vi "Write message.vi"(6 "timeout ms (25000)":i32=25000, 8 "error in":errorcluster, 9 "Value":string, 10 "Message Name":string, 11 "Connection Info":T1) -> (0 "error out":errorcluster, 3 "Connection Info out":T1)   [LabVIEW 2021]
uses:
  Connection Info.ctl
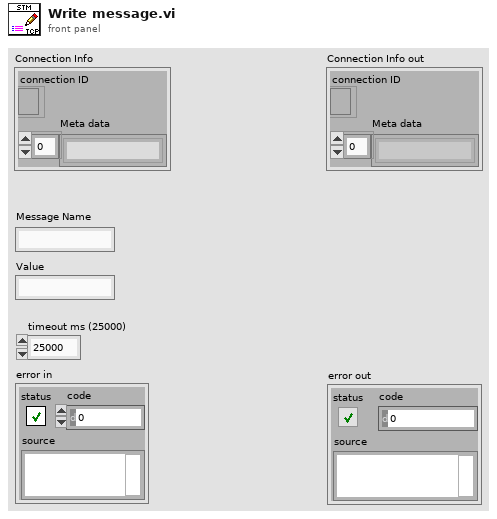
[diagram p1: front panel]
types:
  T1 = typedef "Connection Info.ctl" = cluster{"connection ID":refnum<k5>, "Meta data":string[]}
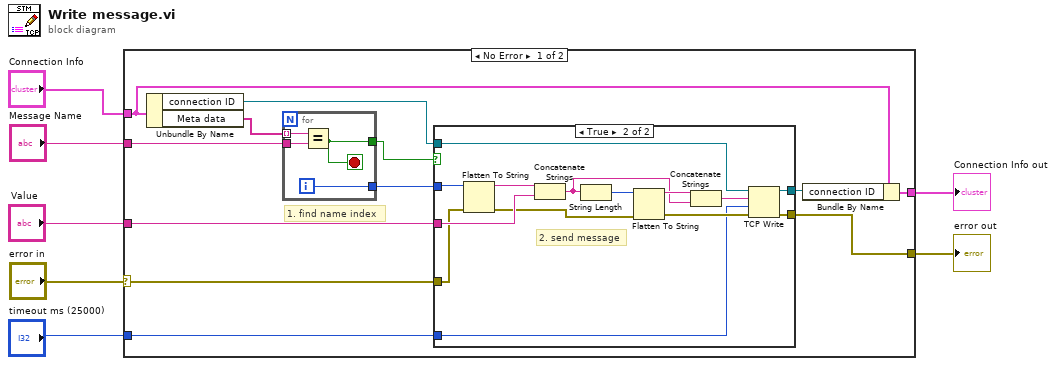
[diagram p0: block diagram]
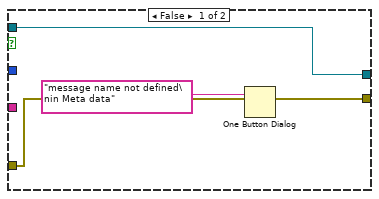
[diagram p2: hidden frame]
diagram:
  n1 = case shown="No Error" "error in" {
    selector: "error in" -> [w14 w42]
    tunnel: "Value" -> [w15 _]
    tunnel: "Message Name" -> [w18 _]
    tunnel: "Connection Info" -> [w9 w41]
    tunnel: "timeout ms (25000)" -> [w12 _]
    tunnel: [w11 w42] -> w3
    tunnel: [w8 w41] -> w1
    frame No Error {
      # "1. find name index"
      n2 = Unbundle By Name(w9) -> ("connection ID"=w13:refnum<k5>, "Meta data"=w19:string[])
      n3 = for {
        tunnel: w19 -> [w40] mode=indexing
        tunnel: w18 -> [w39]
        tunnel: [w38] -> w17
        tunnel: [w37] -> w16
        i -> [w37]
        stop <- w38 stop-if-true
        n4 = Equal?(x=w40, y=w39) -> (x = y?=w38:bool)
      }
      n5 = case shown="True" w17 {
        tunnel: w16 -> [_ w36]
        tunnel: w15 -> [_ w34]
        tunnel: w14 -> [w21 w32]
        tunnel: w13 -> [w22 w28]
        tunnel: w12 -> [_ w25]
        tunnel: [w21 w24] -> w11
        tunnel: [w22 w23] -> w10
        frame False {
          n6 = One Button Dialog(message="message name not defined\nin Meta data" ("source")) -> ()  [unwired: 1 in, 1 out]
        }
        frame True {
          # "2. send message"
          n7 = Flatten To String(anything=w36, error in (no error)=w32) -> (data string=w35:string, error out=w31:errorcluster)  [unwired: 2 in, 1 out]
          n8 = Concatenate Strings(w35, w34) -> (w29:string)
          n9 = String Length(string=w29) -> (length=w33:i32)
          n10 = Flatten To String(anything=w33, error in (no error)=w31) -> (data string=w30:string, error out=w26:errorcluster)  [unwired: 2 in, 1 out]
          n11 = Concatenate Strings(w30, w29) -> (w27:string)
          n12 = TCP Write(connection ID=w28, data in=w27, error in (no error)=w26, 9:w25) -> (connection ID out=w23:refnum<k5>, error out=w24:errorcluster)  [unwired: 1 out]
        }
      }
      n13 = Bundle By Name(cluster=w9, "connection ID"=w10) -> (w8:T1)
    }
    frame Error {
    }
  }
  "error out" <- w3
  "Connection Info out" <- w1
